vi "CPU Usage of Loop.vi"() -> ()   [LabVIEW 2019]
panel:
  in  "stop":bool
  out "y":dbl
  in  "Y-Intercept (b)":dbl
  in  "x":dbl
  in  "Slope (m)":dbl
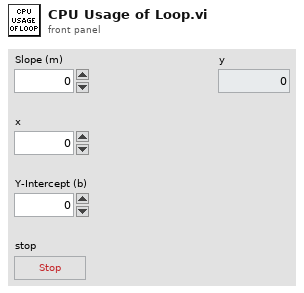
[diagram p1: front panel]
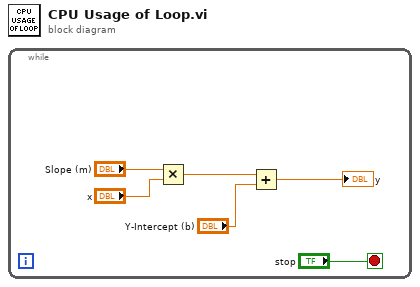
[diagram p0: block diagram]
diagram:
  n1 = while {
    stop <- "stop" stop-if-true
    n2 = Multiply(x="Slope (m)", y="x") -> (x*y=w4:dbl)
    n3 = Add(x=w4, y="Y-Intercept (b)") -> (x+y=→"y":dbl)
  }
